vi "ma_align waveforms (global interval).vi"(0 "Waveform A":waveform(dbl)={"t0"=timestamp(0 s since 1904-01-01), "dt"=0.0, "Y"=[]}, 5 "Waveform B":waveform(dbl)={"t0"=timestamp(0 s since 1904-01-01), "dt"=0.0, "Y"=[]}, 11 "error in":errorcluster, 12 "timestamp difference control":dbl=10.0 format="%.2f") -> (4 "Waveform A out":waveform(dbl), 6 "Waveform B out":waveform(dbl), 15 "error out":errorcluster)   [LabVIEW 2020, in "NI_MAPro.lvlib"]
uses:
  NI_MAPro.lvlib
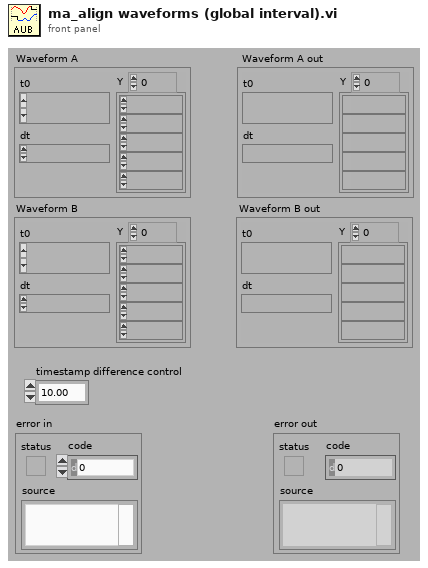
[diagram p1: front panel]
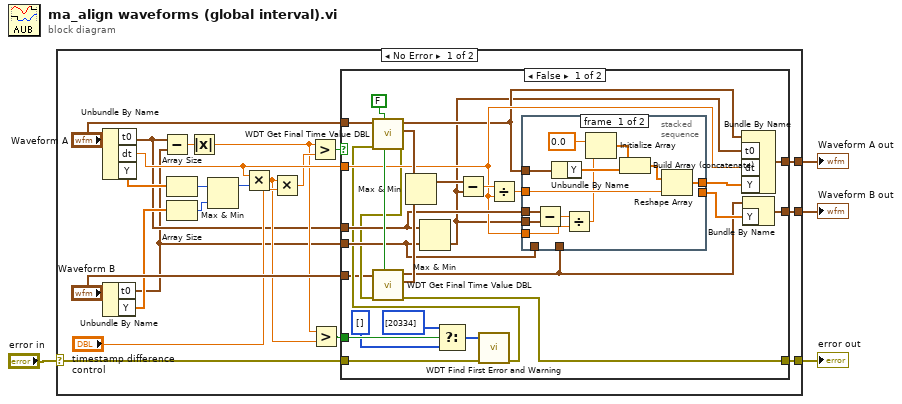
[diagram p0: block diagram]
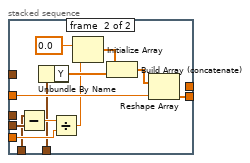
[diagram p2: hidden frame]
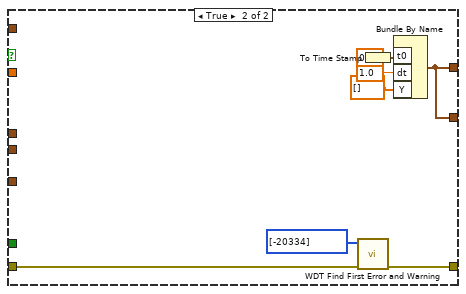
[diagram p3: hidden frame]
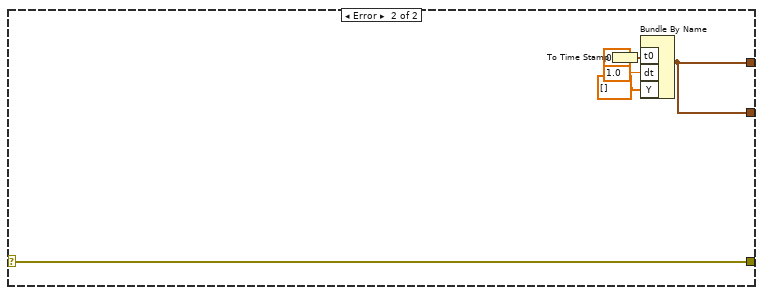
[diagram p4: hidden frame]
diagram:
  n1 = case shown="No Error" "error in" {
    selector: "error in" -> [w13 w89]
    tunnel: [w17 w89] -> w4
    tunnel: [w14 w85] -> w3
    tunnel: [w12 w85] -> w1
    frame No Error {
      n2 = Unbundle By Name("Waveform A") -> ("t0"=w6:timestamp, "dt"=w15:dbl, "Y"=w23:dbl[])
      n3 = Unbundle By Name("Waveform B") -> ("t0"=w5:timestamp, "Y"=w22:dbl[])
      n4 = Subtract(x=w6, y=w5) -> (x-y=w24:dbl)
      n5 = Array Size(array=w23) -> (size(s)=w20:i32)
      n6 = Array Size(array=w22) -> (size(s)=w21:i32)
      n7 = Absolute Value(x=w24) -> (abs(x)=w9:dbl)
      n8 = Max & Min(x=w20, y=w21) -> (max(x,y)=w19:i32)  [unwired: 1 out]
      n9 = Multiply(x=w15, y=w19) -> (x*y=w8:dbl)
      n10 = Multiply(x=w8, y="timestamp difference control") -> (x*y=w10:dbl)
      n11 = Greater?(x=w9, y=w10) -> (0:w18:bool)
      n12 = Greater?(x=w9, y=w8) -> (0:w7:bool)
      n13 = case shown="False" w18 {
        tunnel: [w34 w79] -> w17
        tunnel: "Waveform A" -> [w28 _]
        tunnel: "Waveform B" -> [w30 _]
        tunnel: w6 -> [w45 _]
        tunnel: w5 -> [w44 _]
        tunnel: w15 -> [w43 _]
        tunnel: [w31 w80] -> w14
        tunnel: w13 -> [w39 w78]
        tunnel: [w41 w80] -> w12
        tunnel: w7 -> [w37 _]
        frame False {
          w51 = FALSE ("open interval? (T)")
          n14 = Max & Min(x=w45, y=w44) -> (min(x,y)=w26:timestamp)  [unwired: 1 out]
          n15 = Select(t=i32[] [20334] ("Error Codes"), s=w37, f=i32[] [] ("Error Codes")) -> (s? t:f=w38:i32[])
          n16 = call "WDT Find First Error and Warning.vi"("error in (no error)"=w39, "Error Codes"=w38) -> ("error out"=w36:errorcluster)  [unwired: 4 in, 1 out]
          n17 = call "WDT Get Final Time Value DBL.vi"("open interval? (T)"=w51, "error in (no error)"=w36, "waveform in"=w28) -> ("error out"=w35:errorcluster, "tf"=w50:timestamp, "waveform out"=w27:waveform(dbl))  [unwired: 6 in]
          n18 = call "WDT Get Final Time Value DBL.vi"("open interval? (T)"=w51, "error in (no error)"=w35, "waveform in"=w30) -> ("error out"=w34:errorcluster, "tf"=w49:timestamp, "waveform out"=w29:waveform(dbl))  [unwired: 6 in]
          n19 = Max & Min(x=w50, y=w49) -> (max(x,y)=w48:timestamp)  [unwired: 1 out]
          n20 = Subtract(x=w48, y=w26) -> (x-y=w47:dbl)
          n21 = Divide(x=w47, y=w43) -> (x/y=w46:dbl)
          n22 = stacked-sequence {
            tunnel: w27 -> [w63 _]
            tunnel: w46 -> [w57 w71]
            tunnel: [w58 _] -> w42
            tunnel: [_ w66] -> w40
            tunnel: w45 -> [w56 _]
            tunnel: w26 -> [w55 w70]
            tunnel: w43 -> [w53 w68]
            tunnel: w29 -> [_ w65]
            tunnel: w44 -> [_ w64]
            frame #0 {
              n23 = Subtract(x=w56, y=w55) -> (x-y=w54:dbl)
              n24 = Unbundle By Name(w63) -> ("Y"=w62:dbl[])
              n25 = Divide(x=w54, y=w53) -> (x/y=w52:dbl)
              n26 = Initialize Array(0.0 ("element"), w52) -> (w61:dbl[])
              n27 = Build Array (concatenate)(w61, w62) -> (w59:dbl[])
              n28 = Reshape Array(w59, w57) -> (w58:dbl[])
            }
            frame #1 {
              n29 = Subtract(x=w64, y=w70) -> (x-y=w69:dbl)
              n30 = Unbundle By Name(w65) -> ("Y"=w75:dbl[])
              n31 = Divide(x=w69, y=w68) -> (x/y=w67:dbl)
              n32 = Initialize Array(0.0 ("element"), w67) -> (w74:dbl[])
              n33 = Build Array (concatenate)(w74, w75) -> (w72:dbl[])
              n34 = Reshape Array(w72, w71) -> (w66:dbl[])
            }
          }
          n35 = Bundle By Name(cluster=w27, "t0"=w26, "dt"=w43, "Y"=w42) -> (w31:waveform(dbl))
          n36 = Bundle By Name(cluster=w29, "Y"=w40) -> (w41:waveform(dbl))
        }
        frame True {
          n37 = call "WDT Find First Error and Warning.vi"("error in (no error)"=w78, "Error Codes"=i32[] [-20334]) -> ("error out"=w79:errorcluster)  [unwired: 4 in, 1 out]
          n38 = To Time Stamp(1:0.0 ("t0")) -> (0:w76:timestamp)
          n39 = Bundle By Name("t0"=w76, "dt"=1.0, "Y"=dbl[] []) -> (w80:waveform(dbl))  [unwired: 1 in]
        }
      }
    }
    frame Error {
      n40 = To Time Stamp(1:0.0 ("t0")) -> (0:w84:timestamp)
      n41 = Bundle By Name("t0"=w84, "dt"=1.0, "Y"=dbl[] []) -> (w85:waveform(dbl))  [unwired: 1 in]
    }
  }
  "Waveform A out" <- w3
  "error out" <- w4
  "Waveform B out" <- w1
